vi "Generate Random Queue Name.vi"() -> (3 "Random Queue Name":string)   [LabVIEW 2015, in "Test_Queue.lvclass"]
uses:
  Test_Queue.lvclass
  Global Parameters.vi
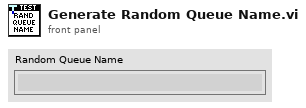
[diagram p1: front panel]
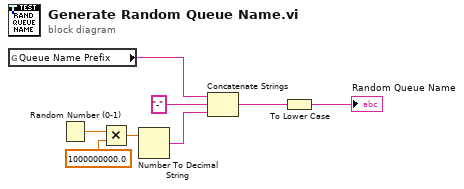
[diagram p0: block diagram]
diagram:
  n1 = global read "Global Parameters.vi" "Queue Name Prefix"() -> (w1:string)
  n2 = Random Number (0-1)() -> (number: 0 to 1=w6:dbl)
  n3 = Multiply(x=w6, y=1000000000.0) -> (x*y=w5:dbl)
  n4 = Number To Decimal String(number=w5) -> (decimal integer string=w8:string)  [unwired: 1 in]
  n5 = Concatenate Strings(w1, "-" ("string"), w8) -> (w3:string)
  n6 = To Lower Case(string=w3) -> (all lower case string=→"Random Queue Name":string)
